vi "GETFIJdll.vi"(8 "error in (no error)":errorcluster, 11 "hmodij":string) -> (0 "error out":errorcluster, 3 "Outputs":T1)   [LabVIEW 2021]
doc: "subroutine GETFIJdll(hmodij, fij, hfij2, hmxrul, hmodij_length, hfij2_length, hmxrul_length)\nRetrieve parameter info for a specified mixing rule.\n\nINPUTS:\nhmodij -- Mixing rule for the binary pair i,j (e.g., LJ6 or KW0) (character*3)\n\nOUTPUTS:\nfij -- Binary mixture parameters (array of dimension nmxpar; currently nmxpar is set to 6). \n The parameters will vary depending on hmodij.\nhfij2 -- description of the binary mixture parameters [character*8 array of dimension nmxpar]for example, for the Lemmon-Jacobsen model (LJ1):\n fij(1) = zeta\n fij(2) = xi\n fij(3) = Fpq\n fij(4) = beta\n fij(5) = gamma\n fij(6) = 'not used'\n\nhmxrul -- Description of the mixing rule (character*255)\nhmodij_length -- length of variable hmodij (default: 3)\nhfij2_length -- length of variable hfij2 (default: 255)\nhmxrul_length -- length of variable hmxrul (default: 255)"
uses:
  REFPROP.dll
panel:
  # "REFPROP-GETFIJdll.vi"
  # "void  GETFIJdll(CStr hmodij, double *fij, CStr hfij2, CStr hmxrul, int32_t hmodij_length, int32_t hfj2_length, int32_t hmxrul_length)"
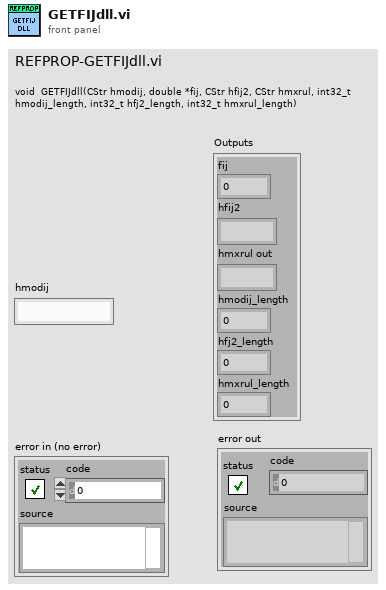
[diagram p1: front panel]
types:
  T1 = cluster{"fij":dbl, "hfij2":string, "hmxrul out":string, "hmodij_length":i32, "hfj2_length":i32, "hmxrul_length":i32}
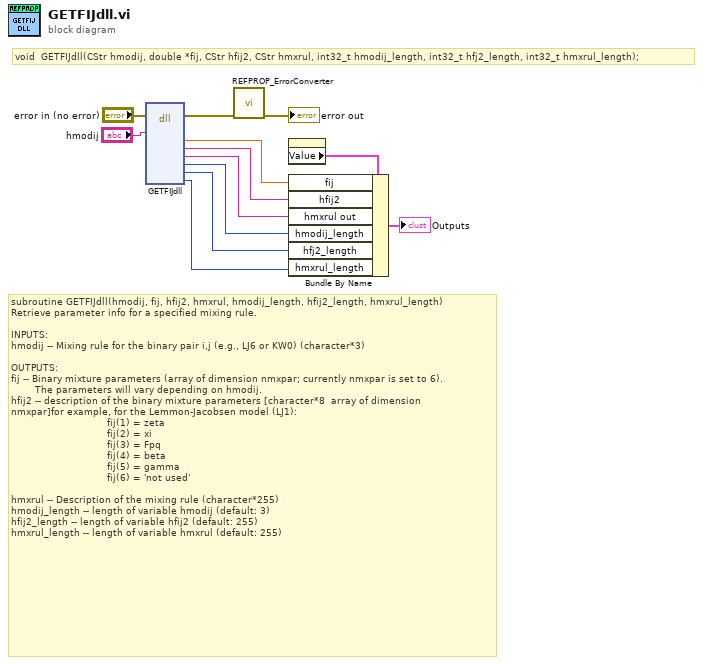
[diagram p0: block diagram]
diagram:
  # "void  GETFIJdll(CStr hmodij, double *fij, CStr hfij2, CStr hmxrul, int32_t hmodij_length, int32_t hfj2_length, int32_t hmxrul_length);"
  # "subroutine GETFIJdll(hmodij, fij, hfij2, hmxrul, hmodij_length, hfij2_length, hmxrul_length)\nRetrieve parameter info for a specified mixing rule.\n\nINPUTS:\nhmodij -- Mixing rule for the binary pair i,j (e.g., LJ6 or KW0) (character*3)\n\nOUTPUTS:\nfij -- Binary mixture parameters (array of dimension nmxpar; currently nmxpar is set to 6). \n        The parameters will vary depending on hmodij.\nhfij2 -- description of the binary mixture parameters [character*8  array of dimension           nmxpar]for example, for the Lemmon-Jacobsen model (LJ1):\n                                fij(1) = zeta\n                                fij(2) = xi\n                                fij(3) = Fpq\n                                fij(4) = beta\n                                fij(5) = gamma\n                                fij(6) = 'not used'\n\nhmxrul -- Description of the mixing rule (character*255)\nhmodij_length -- length of variable hmodij (default: 3)\nhfij2_length -- length of variable hfij2 (default: 255)\nhmxrul_length -- length of variable hmxrul (default: 255)"
  n1 = dll-call lib="C:/Users/lauria/OneDrive - National Institute of Standards and Technology (NIST)/LabVIEW Projects/7 REFPROP/REFPROP-wrappers-master/REFPROP-wrappers-master/wrappers/Labview/REFPROP/REFPROP.*" fn="GETFIJdll"(error in="error in (no error)", "hmodij"="hmodij") -> (error out=w11:errorcluster, "fij"=w2:dbl, "hfij2"=w3:string, "hmxrul"=w4:string, "hmodij_length"=w5:i32, "hfj2_length"=w6:i32, "hmxrul_length"=w7:i32)  [unwired: 10 in, 1 out]
  n2 = call "REFPROP_ErrorConverter.vi"("error in (no error)"=w11) -> ("error out"=→"error out":errorcluster)  [unwired: 10 in]
  n3 = property on="Outputs" class="Clust (strict)"() -> ("Value"=w8:T1)  [unwired: 2 in, 2 out]
  n4 = Bundle By Name(cluster=w8, "fij"=w2, "hfij2"=w3, "hmxrul out"=w4, "hmodij_length"=w5, "hfj2_length"=w6, "hmxrul_length"=w7) -> (→"Outputs":T1)
